vi "UI_Resize.vi"(8 "error in (no error)":errorcluster, 11 "DualScreen in":refnum<class "DualScreen.lvclass">) -> (0 "error out":errorcluster, 3 "DualScreen out":refnum<class "DualScreen.lvclass">)   [LabVIEW 2020, in "DualScreen.lvlib" / "DualScreen.lvclass"]
uses:
  DualScreen.lvclass
  D:/Projets/STEP AT/Bahamut/support/UI_Actor.lvlibp/UI_Actor/UI_Actor.lvclass
  DualScreen.lvclass/DualScreen.ctl
  support/UI_Actor.lvlibp/UI_Actor/Read Nested UIA Qs.vi
  support/Actor Framework.lvlibp/1abvi3w/vi.lib/ActorFramework/Message Enqueuer/Message Enqueuer.lvclass
  support/UI_Actor.lvlibp/UI_Actor Messages/UI_Resize Msg/UI_Resize Msg.lvclass
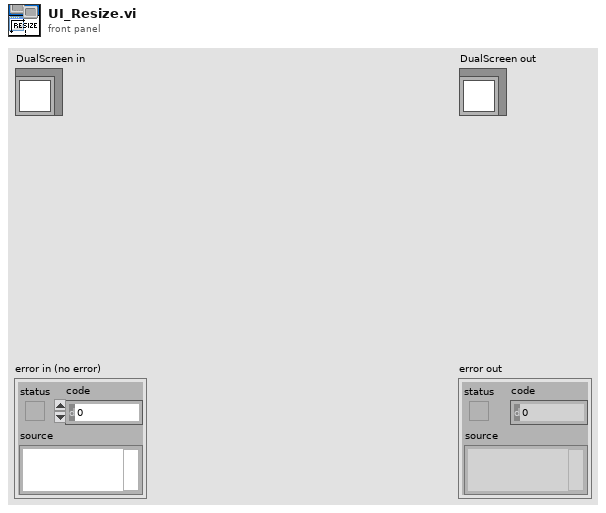
[diagram p1: front panel]
types:
  T1 = enum16{"Sticks Top/Left", "Sticks Bottom/Right", "Proportional"}
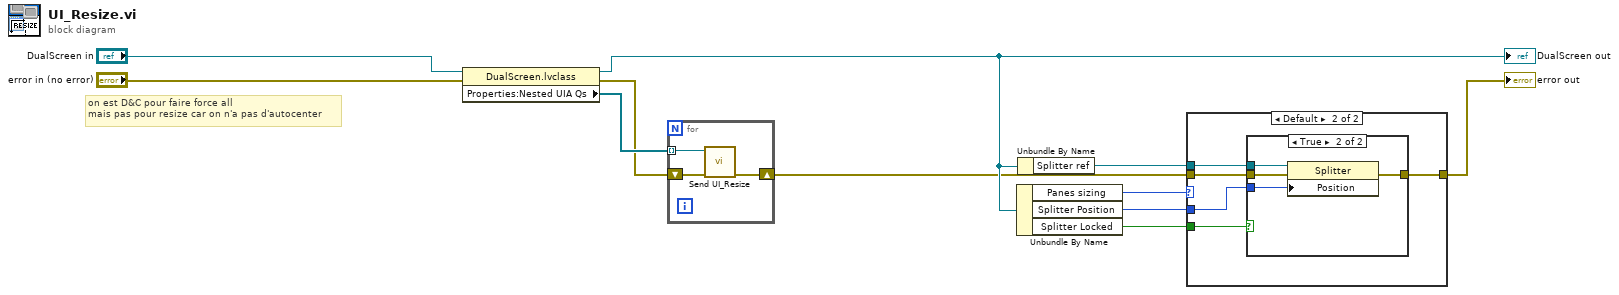
[diagram p0: block diagram]
diagram:
  # "on est D&C pour faire force all\nmais pas pour resize car on n'a pas d'autocenter"
  n1 = property class="DualScreen.lvclass"(reference="DualScreen in", error in="error in (no error)") -> (reference out=w7:refnum<class "DualScreen.lvclass">, error out=w10:errorcluster, "Properties:Nested UIA Qs"=w11:refnum<class "Message Enqueuer.lvclass">[])
  "DualScreen out" <- w7
  n2 = for {
    tunnel: w11 -> [w14] mode=indexing
    shift-right: [w12] -> w3
    shift-left: w10 -> [w13]
    n3 = call "Send UI_Resize.vi"("error in (no error)"=w13, "Message Enqueuer"=w14) -> ("error out"=w12:errorcluster)  [unwired: 8 in, 1 out]
  }
  n4 = Unbundle By Name(w7) -> ("Panes sizing"=w5:T1, "Splitter Position"=w4:i32, "Splitter Locked"=w1:bool)
  n5 = Unbundle By Name(w7) -> ("Splitter ref"=w6:refnum<vi>)
  n6 = case shown="Default" w5 {
    tunnel: w6 -> [_ w20]
    tunnel: w3 -> [w15 w19]
    tunnel: w4 -> [_ w18]
    tunnel: [w15 w17] -> w2
    tunnel: w1 -> [_ w16]
    frame "Proportional" {
    }
    frame Default {
      n7 = case shown="True" w16 {
        tunnel: w20 -> [_ w25]
        tunnel: w19 -> [w21 w24]
        tunnel: w18 -> [_ w23]
        tunnel: [w21 w22] -> w17
        frame False {
        }
        frame True {
          n8 = property class="Splitter"(reference=w25, error in=w24, "Position"=w23) -> (error out=w22:errorcluster)  [unwired: 1 out]
        }
      }
    }
  }
  "error out" <- w2
